vi "Print VI to Printer using VI Server Core.vi"(1 "error in":errorcluster, 2 "layout options":T2 {"page header options"."page headers (unchanged)" items=["Unchanged", "Include page headers", "Do not include page headers"]; "printer options"."color or monochrome (unchanged)" items=["Unchanged", "Color/grayscale", "Monochrome"]; "printer options"."printing method (unchanged)" items=["Unchanged", "Standard", "PostScript", "Bitmap"]; "panel scaling for page (unchanged)" items=["Unchanged", "No Scaling", "Scale front panel to fit"]; "orientation (unchanged)" items=["Unchanged", "portrait", "landscape"]; "margins"."measurement system (default)" items=["Default", "US", "Metric"]; "margins"."margins (1.00)"."right" format="%.2f"; "margins"."margins (1.00)"."bottom" format="%.2f"; "margins"."margins (1.00)"."top" format="%.2f"; "margins"."margins (1.00)"."left" format="%.2f"}, 3 "Format":T1=2 items=["Complete front panel", "Visible portion of front panel", "Icon, description, panel and diagram", "Documentation: Using the panel", "Documentation: Using as a subVI", "Documentation: Complete", "Documentation: Custom"], 4 "VI reference":refnum<vi>) -> (0 "error out":errorcluster)   [LabVIEW 2020, in "NI_ReportGenerationCore.lvlib"]
uses:
  <vilib>/Utility/NIReport.llb/NI_ReportGenerationCore.lvlib
  <vilib>/printing/EasyPrintingControls.llb/layout_options.ctl
  <vilib>/printing/EasyPrintingControls.llb/orientation.ctl
  <vilib>/printing/EasyPrintingControls.llb/panel_scaling_for_page.ctl
  <vilib>/printing/EasyPrintingControls.llb/margins.ctl
  <vilib>/printing/EasyPrintingControls.llb/margin_values.ctl
  <vilib>/printing/EasyPrintingControls.llb/measurement_system.ctl
  <vilib>/printing/EasyPrintingControls.llb/printer_options.ctl
  <vilib>/printing/EasyPrintingControls.llb/printing_method.ctl
  <vilib>/printing/EasyPrintingControls.llb/color_or_monochrome.ctl
  <vilib>/printing/EasyPrintingControls.llb/page_header_options.ctl
  <vilib>/printing/EasyPrintingControls.llb/page_headers.ctl
  <vilib>/printing/EasyPrintingControls.llb/page_header_content_options.ctl
  <vilib>/printing/EasyPrintingControls.llb/contents.ctl
  <vilib>/printing/EasyPrintingControls.llb/page_headers_ENUM.ctl
  <vilib>/printing/EasyPrintingControls.llb/contents_ENUM.ctl
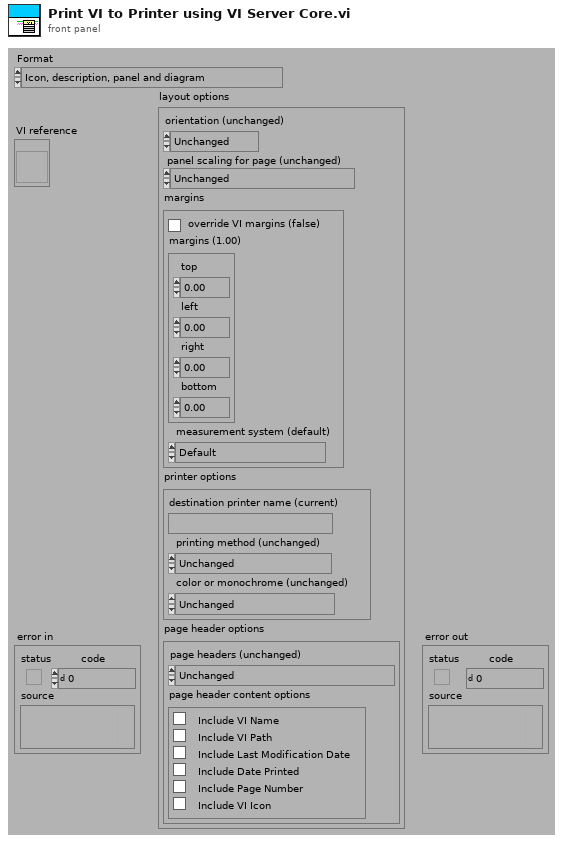
[diagram p1: front panel]
types:
  T1 = typedef "NI_ReportGenerationCore.lvlib/contents.ctl" = u16
  T2 = typedef "NI_ReportGenerationCore.lvlib/layout_options.ctl" = cluster{"orientation (unchanged)":T3, "panel scaling for page (unchanged)":T4, "margins":T5, "printer options":T8, "page header options":T11}
  T3 = typedef "NI_ReportGenerationCore.lvlib/orientation.ctl" = u16
  T4 = typedef "NI_ReportGenerationCore.lvlib/panel_scaling_for_page.ctl" = u16
  T5 = typedef "NI_ReportGenerationCore.lvlib/margins.ctl" = cluster{"override VI margins (false)":bool, "margins (1.00)":T6, "measurement system (default)":T7}
  T6 = typedef "NI_ReportGenerationCore.lvlib/margin_values.ctl" = cluster{"top":dbl, "left":dbl, "right":dbl, "bottom":dbl}
  T7 = typedef "NI_ReportGenerationCore.lvlib/measurement_system.ctl" = u16
  T8 = typedef "NI_ReportGenerationCore.lvlib/printer_options.ctl" = cluster{"destination printer name (current)":string, "printing method (unchanged)":T9, "color or monochrome (unchanged)":T10}
  T9 = typedef "NI_ReportGenerationCore.lvlib/printing_method.ctl" = u16
  T10 = typedef "NI_ReportGenerationCore.lvlib/color_or_monochrome.ctl" = u16
  T11 = typedef "NI_ReportGenerationCore.lvlib/page_header_options.ctl" = cluster{"page headers (unchanged)":T12, "page header content options":T13}
  T12 = typedef "NI_ReportGenerationCore.lvlib/page_headers.ctl" = u16
  T13 = typedef "NI_ReportGenerationCore.lvlib/page_header_content_options.ctl" = cluster{"Include VI Name":bool, "Include VI Path":bool, "Include Last Modification Date":bool, "Include Date Printed":bool, "Include Page Number":bool, "Include VI Icon":bool}
  T14 = typedef "NI_ReportGenerationCore.lvlib/contents_ENUM.ctl" = enum16{"Complete front panel", "Visible portion of front panel", "Icon, description, panel and diagram", "Documentation: Using the panel", "Documentation: Using as a subVI", "Documentation: Complete", "Documentation: Custom"}
  T15 = typedef "NI_ReportGenerationCore.lvlib/page_headers_ENUM.ctl" = enum16{"Unchanged", "Include page headers", "Do not include page headers"}
  T16 = enum32{"Custom", "Standard", "Using Panel", "Using SubVI", "Complete"}
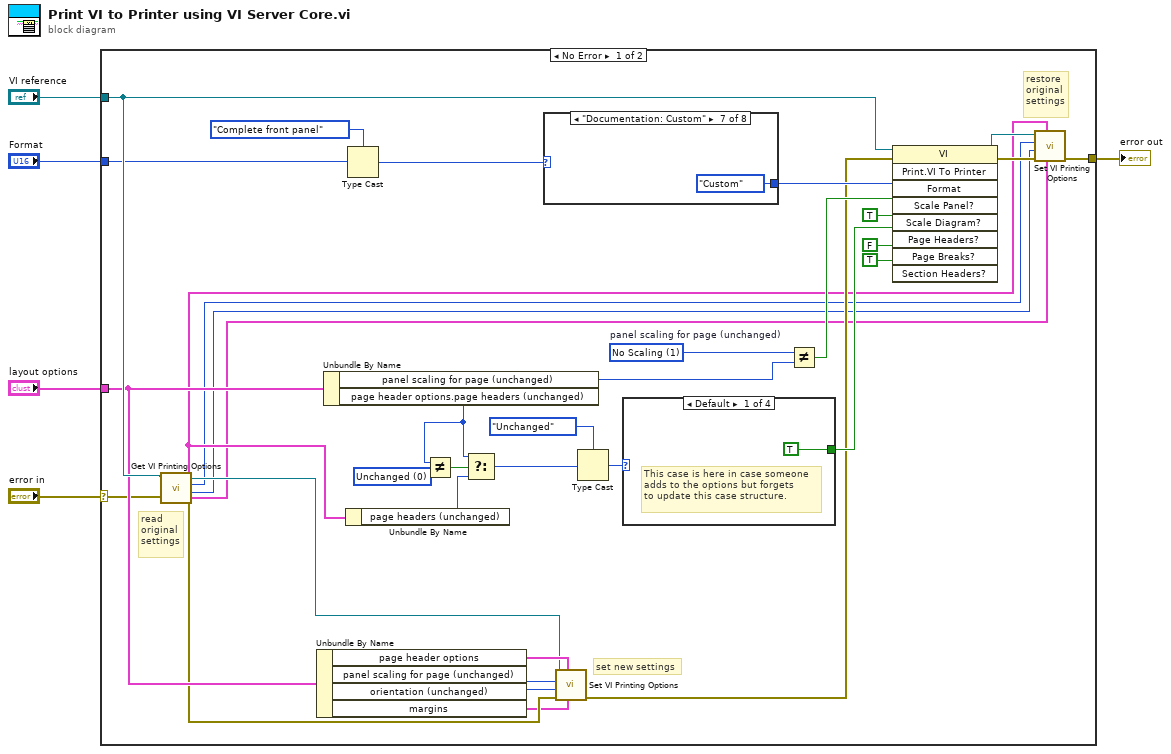
[diagram p0: block diagram]
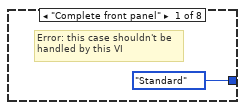
[diagram p2: hidden frame]
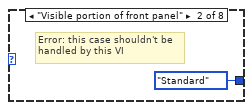
[diagram p3: hidden frame]
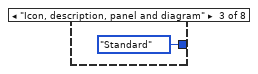
[diagram p4: hidden frame]
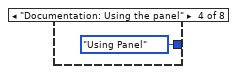
[diagram p5: hidden frame]
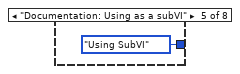
[diagram p6: hidden frame]
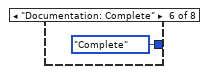
[diagram p7: hidden frame]
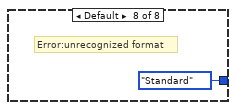
[diagram p8: hidden frame]
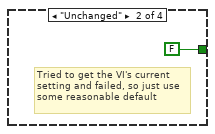
[diagram p9: hidden frame]
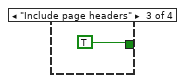
[diagram p10: hidden frame]
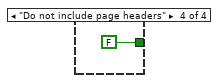
[diagram p11: hidden frame]
diagram:
  n1 = case shown="No Error" "error in" {
    selector: "error in" -> [w6 w53]
    tunnel: "VI reference" -> [w32 _]
    tunnel: "Format" -> [w27 _]
    tunnel: "layout options" -> [w21 _]
    tunnel: [w12 w53] -> w2
    frame No Error {
      w22 = T4 1 items=["Unchanged", "No Scaling", "Scale front panel to fit"]  # panel scaling for page (unchanged)
      w33 = T12 0 items=["Unchanged", "Include page headers", "Do not include page headers"] ("page header options.page headers (unchanged)")
      # "restore\noriginal\nsettings"
      # "set new settings"
      # "read\noriginal\nsettings"
      n2 = call <vilib>:"Get VI Printing Options.vi"("error in (no error)"=w6, "VI Refnum"=w32) -> ("error out"=w16:errorcluster, "orientation (unchanged)"=w8:T3, "panel scaling for page (unchanged)"=w9:T4, "VI Refnum out"=w19:refnum<vi>, "margins"=w7:T5, "page header options"=w10:T11)  [unwired: 4 in]
      n3 = Unbundle By Name(w21) -> ("page header options"=w20:T11, "panel scaling for page (unchanged)"=w18:T4, "orientation (unchanged)"=w17:T3, "margins"=w15:T5)
      n4 = Unbundle By Name(w21) -> ("panel scaling for page (unchanged)"=w23:T4, "page header options.page headers (unchanged)"=w30:T12)
      n5 = Unbundle By Name(w10) -> ("page headers (unchanged)"=w28:T12)
      n6 = Type Cast(type=contents_ENUM."Complete front panel" ("Enum"), x=w27) -> (*(type *) &x=w25:T14)
      n7 = Not Equal?(x=w30, y=w33) -> (x != y?=w31:bool)
      n8 = Select(t=w30, s=w31, f=w28) -> (s? t:f=w29:T12)
      n9 = case shown="\"Documentation: Custom\"" w25 {
        tunnel: [T16."Standard" ("Format") T16."Standard" ("Format") T16."Standard" ("Format") T16."Using Panel" ("Format") T16."Using SubVI" ("Format") T16."Complete" ("Format") T16."Custom" ("Format") T16."Standard" ("Format")] -> w24
        frame "Complete front panel" {
          # "Error: this case shouldn't be\nhandled by this VI"
        }
        frame "Visible portion of front panel" {
          # "Error: this case shouldn't be\nhandled by this VI"
        }
        frame "Icon, description, panel and diagram" {
        }
        frame "Documentation: Using the panel" {
        }
        frame "Documentation: Using as a subVI" {
        }
        frame "Documentation: Complete" {
        }
        frame "Documentation: Custom" {
        }
        frame Default {
          # "Error:unrecognized format"
        }
      }
      n10 = call <vilib>:"Set VI Printing Options.vi"("margins"=w15, "page header options"=w20, "error in (no error)"=w16, "orientation (unchanged)"=w17, "panel scaling for page (unchanged)"=w18, "VI Refnum"=w19) -> ("error out"=w14:errorcluster)  [unwired: 4 in, 1 out]
      n11 = Type Cast(type=page_headers_ENUM."Unchanged" ("page headers (unchanged)"), x=w29) -> (*(type *) &x=w36:T15)
      n12 = case shown="Default" w36 {
        tunnel: [TRUE FALSE TRUE FALSE] -> w34
        frame Default {
          # "This case is here in case someone\nadds to the options but forgets\nto update this case structure."
        }
        frame "Unchanged" {
          # "Tried to get the VI's current\nsetting and failed, so just use\nsome reasonable default"
        }
        frame "Include page headers" {
        }
        frame "Do not include page headers" {
        }
      }
      n13 = Not Equal?(x=w22, y=w23) -> (x != y?=w35:bool)
      n14 = invoke class="VI" method="Print.VI To Printer"(reference=w32, error in=w14, "Format"=w24, "Scale Panel?"=w35, "Scale Diagram?"=TRUE, "Page Headers?"=w34, "Page Breaks?"=FALSE, "Section Headers?"=TRUE) -> (reference out=w11:refnum<vi>, error out=w13:errorcluster)  [unwired: 1 in, 7 out]
      n15 = call <vilib>:"Set VI Printing Options.vi"("margins"=w7, "page header options"=w10, "error in (no error)"=w13, "orientation (unchanged)"=w8, "panel scaling for page (unchanged)"=w9, "VI Refnum"=w11) -> ("error out"=w12:errorcluster)  [unwired: 4 in, 1 out]
    }
    frame Error {
    }
  }
  "error out" <- w2
